vi "Ball Target Loop.vi"(0 "Camera List":string[](array[string]), 1 "Instance":i32) -> ()   [LabVIEW 2025]
uses:
  Camera Set Up/Ctrl/White Balance.ctl
  State Machine/Ball States.ctl
  State Machine/Ball Main CLuster.ctl
  <vilib>/vision/Image Controls.llb/IMAQ Image.ctl
  Camera Set Up/Event/Event Setup Types.ctl
  Steam Type.ctl
  <vilib>/Utility/config.llb/Read Key (String).vi
  <vilib>/Utility/config.llb/Write Key (String).vi
  <vilib>/Utility/config.llb/NI_LVConfig.lvlib
  <vilib>/vision/NI_Vision_Development_Module.lvlib
panel:
  in  "Running":bool
  in  "Timeout":u32
  in  "Main":T1(tab)
  out "Image":T2(plugin-control)
  out "Camera Name":string="cam0"
  out "Fule Distance":dbl[](array[numeric]) caption="Distance" format="%.1f"
  out "Fule Angle":dbl[](array[numeric]) caption="Angle" format="%.1f"
  in  "Settings":bool
  in  "Save":bool
  in  "Tools":bool
  out "Ball Fps":dbl format="%#.0f"
  in  "Color Range":T3={"Hue"={103, 151}, "Sat"={217, 255}, "Val"={201, 249}} {"Val" scale format="%#.0f"; "Sat" scale format="%#.0f"; "Hue" scale=0.0..255.0 scale format="%#.0f"}
  in  "Home":bool
  in  "Ball Diameter (in)":dbl=16.0
  in  "FOV":dbl=68.5
  out "Mask":T2(plugin-control)
  in  "Score Threshold %":dbl=80.0
  out "Camera Name 2":string="cam0"
  in  "VideoMode":u16(ring)=20 items=["160x120 MJPG 30.00fps", "160x120 YUY2 30.00fps", "176x144 MJPG 30.00fps", "176x144 YUY2 30.00fps", "320x240 MJPG 30.00fps", "320x240 YUY2 30.00fps", "352x288 MJPG 30.00fps", "352x288 YUY2 30.00fps", "416x240 MJPG 30.00fps", "424x240 YUY2 30.00fps", "640x360 MJPG 30.00fps", "640x360 YUY2 30.00fps", "640x480 MJPG 30.00fps", "640x480 YUY2 30.00fps", "800x448 MJPG 30.00fps", "800x448 YUY2 20.00fps", "800x600 MJPG 30.00fps", "800x600 YUY2 15.00fps", "960x544 MJPG 30.00fps", "960x544 YUY2 15.00fps", "1280x720 MJPG 30.00fps", "1280x720 YUY2 10.00fps", "1280x800 YUY2 10.00fps"]
  in  "Saturation":i32(slide)=50 min=1 max=100 scale=0.0..100.0
  in  "Hue":i32(slide)=50 min=1 max=100 scale=0.0..100.0
  in  "Gamma":i32(slide)=50 min=1 max=100 scale=0.0..100.0
  in  "Exposure":dbl(slide)=2.0 min=1.0 max=5.0 scale=0.0..5.0
  in  "Contrast":i32(slide)=50 min=1 max=100 scale=0.0..100.0
  in  "Sharpness":i32(slide)=50 min=1 max=100 scale=0.0..100.0
  in  "White Balance":T4=enum."Hold current"
  in  "Gain":i32(slide)=50 min=1 max=100 scale=0.0..100.0
  in  "Brightness":i32(slide)=50 min=1 max=100 scale=0.0..100.0
  in  "Save 2":bool caption="Save"
  out "Width":u32=640
  out "Height":u32=360
  out "Camera Name 3":string="cam0"
  in  "Home 2":bool caption="Home"
  out "Camera Image":T2(plugin-control)
  out "Data to Send":dbl[][](array[numeric])
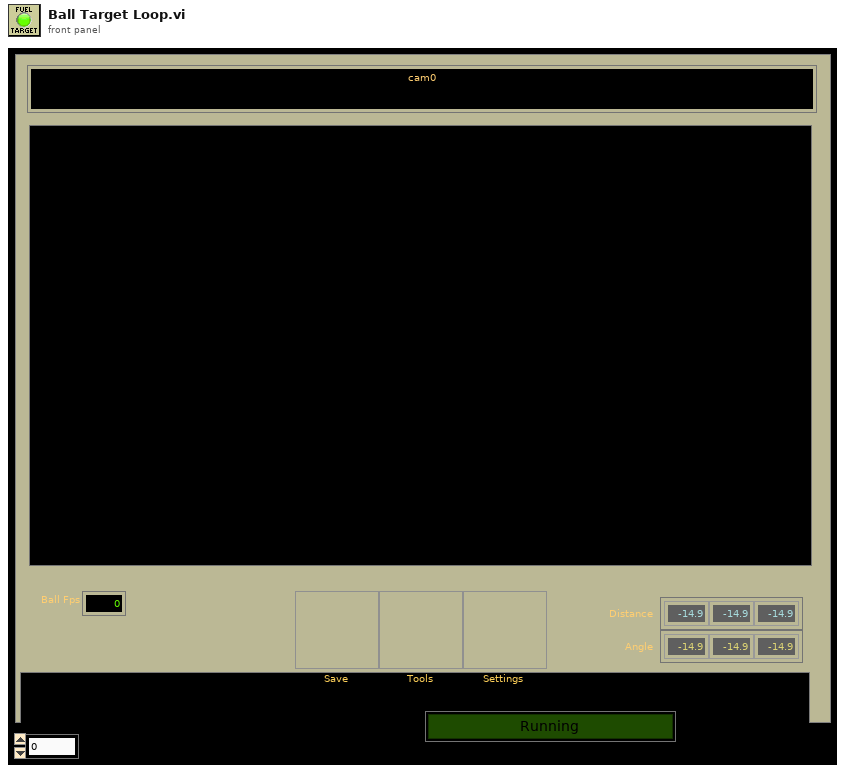
[diagram p1: front panel]
types:
  T1 = enum32{"Main", "Threshold", "Camera Settings", "Misc"}
  T2 = typedef "IMAQ Image.ctl" = refnum<image>
  T3 = cluster{"Hue":cluster{i64, i64}, "Sat":cluster{i64, i64}, "Val":cluster{i64, i64}}
  T4 = typedef "White Balance.ctl" = enum16{"Auto", "Fixed indoor", "Fixed outdoor 1", "Fixed outdoor 2", "Fixed fluorescent 1", "Fixed fluorescent 2", "Hold current", "Custom"}
  T5 = typedef "Ball Main CLuster.ctl" = cluster{"Ball FIFO":T6[], "Camera Name":string, "Ball path":path, "Control Ref's":refnum<vi>[], "Mask Image":T2, "Main Image":T2, "Algae Color Range":cluster{"Hue":cluster{dbl, dbl}, "Sat":cluster{dbl, dbl}, "Val":cluster{dbl, dbl}}, "EDIT Settings":bool, "Camera Number":i32}
  T6 = typedef "Ball States.ctl" = enum16{"Message Dispatcher", "INI", "Open", "Save", "Exit"}
  T7 = typedef "Particle Parameters" = i32
  T8 = typedef "Event Setup Types.ctl" = enum16{"Default", "Camera Loop Started", "GreyScale", "Reset Camera Settings", "Reset Team Number", "Save Data", "Setting Changed", "Update Video Mode", "Video Mode Changed", "Exit"}
  T9 = cluster{"Hue":cluster{dbl, dbl}, "Sat":cluster{dbl, dbl}, "Val":cluster{dbl, dbl}}
  T10 = cluster{"Hue":cluster{i64, dbl}, "Sat":cluster{i64, dbl}, "Val":cluster{i64, dbl}}
  T11 = typedef "Target Fields.ctl" = cluster{"diameter points":cluster{"first point":cluster{"x":dbl, "y":dbl}, "projected point":cluster{"x":dbl, "y":dbl}}, "normalized center":cluster{"x":dbl, "y":dbl}, "Overall Score":dbl, "Area Score":dbl, "Moment Score":dbl, "Aspect Score":dbl, "Distance (ft)":dbl, "Upper Goal":bool}
  T12 = cluster{cluster{"Lower":dbl, "Upper":dbl}, cluster{"Lower":dbl, "Upper":dbl}, cluster{"Lower":dbl, "Upper":dbl}}
  T13 = typedef "Image Type" = u32
  T14 = typedef "NI_LVConfig.lvlib/Config Data RefNum.ctl" = refnum<k1>
  T15 = typedef "Steam Type.ctl" = enum8{"Unknown", "Apriltag", "Fuel", "Other"}
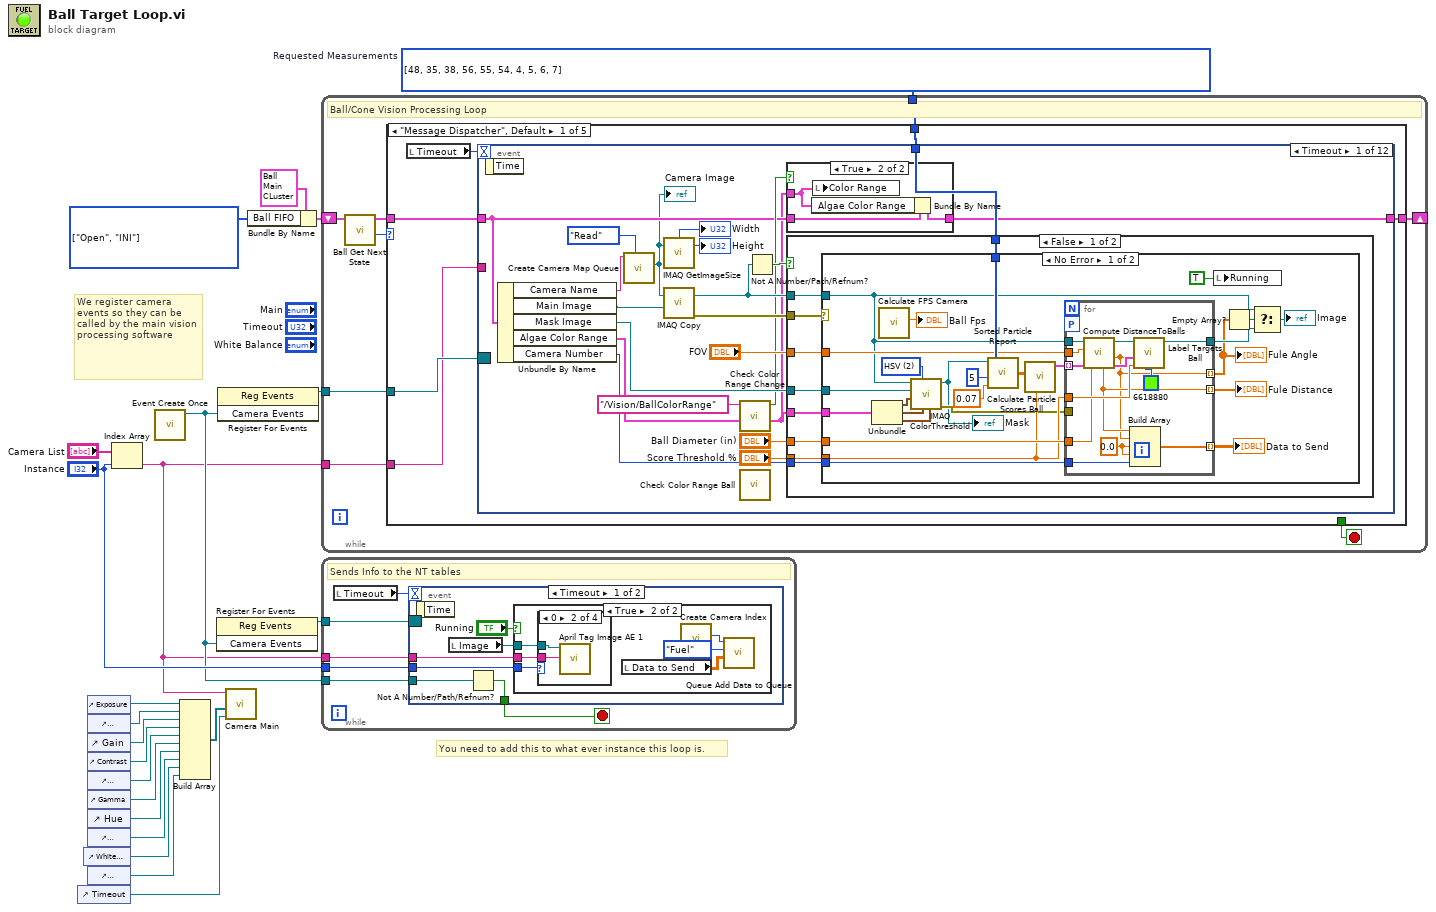
[diagram p0: block diagram]
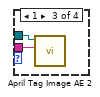
[diagram p4: hidden frame]
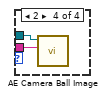
[diagram p5: hidden frame]
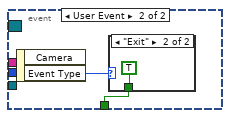
[diagram p6: hidden frame]
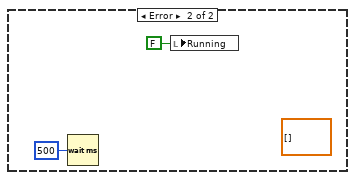
[diagram p9: hidden frame]
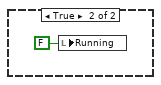
[diagram p10: hidden frame]
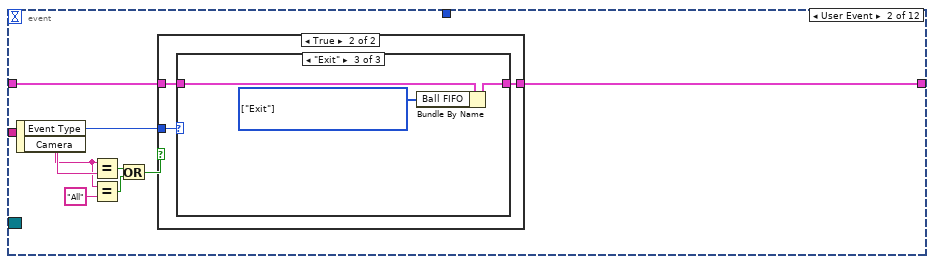
[diagram p11: hidden frame]
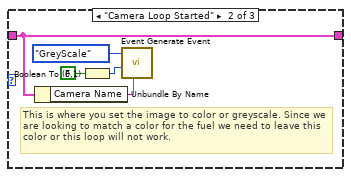
[diagram p14: hidden frame]
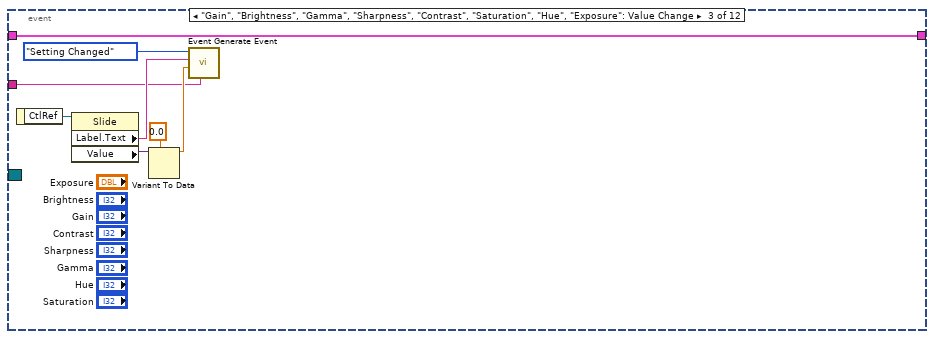
[diagram p15: hidden frame]
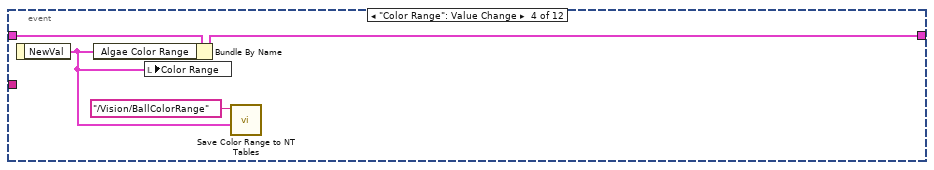
[diagram p16: hidden frame]
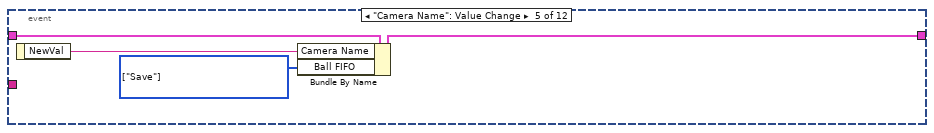
[diagram p17: hidden frame]
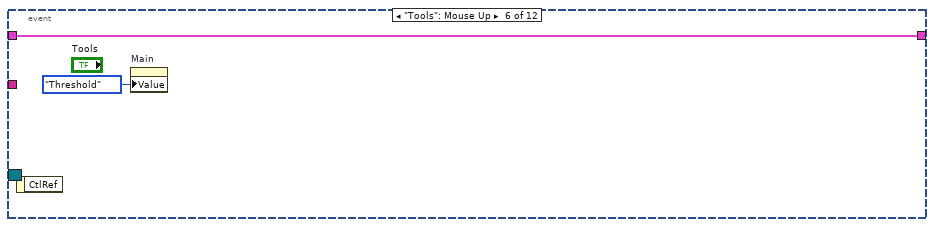
[diagram p18: hidden frame]
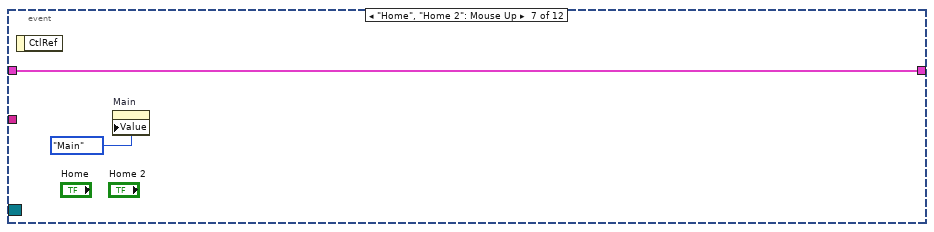
[diagram p19: hidden frame]
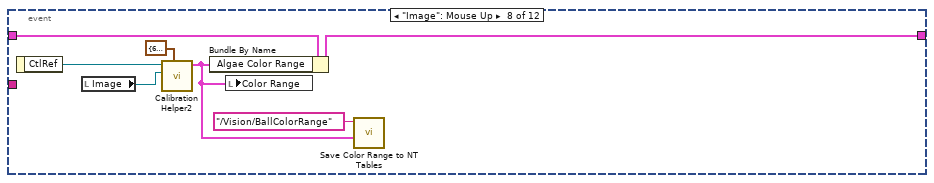
[diagram p20: hidden frame]
diagram:
  w19 = T6[] [enum."Open", enum."INI"] items=["Message Dispatcher", "INI", "Open", "Save", "Exit"] ("Ball FIFO")
  w21 = T7[] [48, 35, 38, 56, 55, 54, 4, 5, 6, 7] items=["Center of Mass X", "Center of Mass Y", "First Pixel X", "First Pixel Y", "Bounding Rect Left", "Bounding Rect Top", "Bounding Rect Right", "Bounding Rect Bottom", "Max Feret Diameter Start X", "Max Feret Diameter Start Y", "Max Feret Diameter End X", "Max Feret Diameter End Y", "Max Horiz. Segment Length Left", "Max Horiz. Segment Length Right", "Max Horiz. Segment Length Row", "-", "Bounding Rect Width", "Bounding Rect Height", "Bounding Rect Diagonal", "Perimeter", "Convex Hull Perimeter", "Holes' Perimeter", "Max Feret Diameter", "Equivalent Ellipse Major Axis", "Equivalent Ellipse Minor Axis", "Equivalent Ellipse Minor Axis (Feret)", "Equivalent Rect Long Side", "Equivalent Rect Short Side", "Equivalent Rect Diagonal", "Equivalent Rect Short Side (Feret)", "Average Horiz. Segment Length", "Average Vert. Segment Length", "Hydraulic Radius", "Waddel Disk Diameter", "-", "Area", "Holes' Area", "Particle & Holes' Area", "Convex Hull Area", "Image Area", "-", "Number of Holes", "Number of Horiz. Segments", "Number of Vert. Segments", "-", "Orientation", "Max Feret Diameter Orientation", "-", "% Area/Image Area", "% Area/(Particle & Holes' Area)", "Ratio of Equivalent Ellipse Axes", "Ratio of Equivalent Rect Sides", "-", "Elongation Factor", "Compactness Factor", "Heywood Circularity Factor", "Type Factor", "-", "Sum X", "Sum Y", "Sum XX", "Sum XY", "Sum YY", "Sum XXX", "Sum XXY", "Sum XYY", "Sum YYY", "-", "Moment of Inertia XX", "Moment of Inertia XY", "Moment of Inertia YY", "Moment of Inertia XXX", "Moment of Inertia XXY", "Moment of Inertia XYY", "Moment of Inertia YYY", "Norm. Moment of Inertia XX", "Norm. Moment of Inertia XY", "Norm. Moment of Inertia YY", "Norm. Moment of Inertia XXX", "Norm. Moment of Inertia XXY", "Norm. Moment of Inertia XYY", "Norm. Moment of Inertia YYY", "Hu Moment 1", "Hu Moment 2", "Hu Moment 3", "Hu Moment 4", "Hu Moment 5", "Hu Moment 6", "Hu Moment 7"]  # Requested Measurements
  # "You need to add this to what ever instance this loop is."
  # "We register camera events so they can be called by the main vision processing software"
  n1 = control-ref of="Timeout"() -> (w4:refnum<vi>)
  n2 = control-ref of="White Balance"() -> (w3:refnum<vi>)
  n3 = control-ref of="Exposure"() -> (w13:refnum<vi>)
  n4 = control-ref of="Brightness"() -> (w12:refnum<vi>)
  n5 = control-ref of="Gain"() -> (w11:refnum<vi>)
  n6 = control-ref of="Contrast"() -> (w10:refnum<vi>)
  n7 = control-ref of="Sharpness"() -> (w9:refnum<vi>)
  n8 = control-ref of="Gamma"() -> (w8:refnum<vi>)
  n9 = control-ref of="Hue"() -> (w7:refnum<vi>)
  n10 = control-ref of="Saturation"() -> (w6:refnum<vi>)
  n11 = control-ref of="VideoMode"() -> (w2:refnum<vi>)
  n12 = Index Array(array="Camera List", index="Instance") -> (element=w5:string)
  n13 = call "Event Create Once.vi"() -> ("Camera Events"=w14:refnum<user-event>)  [unwired: 10 in, 1 out]
  n14 = Build Array(w13, w12, w11, w10, w9, w8, w7, w6, w3, w2) -> (w1:refnum<vi>[])
  n15 = register-events(w14) -> (reference out=w15:refnum<event-registration>)  [unwired: 2 in, 1 out]
  n16 = register-events(w14) -> (reference out=w22:refnum<event-registration>)  [unwired: 2 in, 1 out]
  n17 = call "Camera Main.vi"("Timeout 2"=w4, "Main Open and Save Ctrls Ref"=w1, "Camera"=w5) -> ()  [unwired: 9 in]
  n18 = Bundle By Name(cluster=T5 {"Ball FIFO"=[], "Camera Name"="", "Ball path"=path "", "Control Ref's"=[], "Mask Image"=refnum, "Main Image"=refnum, "Algae Color Range"={"Hue"={21.620689392089844, 69.62068939208984}, "Sat"={66.41378784179688, 255.0}, "Val"={96.0, 255.0}}, "EDIT Settings"=FALSE, "Camera Number"=5} ("Ball Main Cluster in"), "Ball FIFO"=w19) -> (w20:T5)
  n19 = while {
    tunnel: w21 -> [w30]
    tunnel: w22 -> [w29]
    shift-right: [w24] -> _
    shift-left: w20 -> [w27]
    tunnel: w5 -> [w23]
    stop <- w28 stop-if-true
    # "Ball/Cone Vision Processing Loop"
    n20 = call "Ball Get Next State.vi"("Ball Main Cluster in"=w27) -> ("Next State"=w26:T6, "Ball Main Cluster out"=w25:T5)  [unwired: 9 in]
    n21 = case shown="\"Message Dispatcher\", Default" w26 {
      tunnel: w30 -> [w36 _ _ _ _]
      tunnel: w29 -> [w35 _ _ _ _]
      tunnel: [_ _ _ _ TRUE] -> w28
      tunnel: w25 -> [w33 w191 w205 w258 w275]
      tunnel: [w34 w190 w203 w258 w275] -> w24
      tunnel: w23 -> [w31 w175 _ _ _]
      frame "Message Dispatcher", Default {
        n22 = local read "Timeout"() -> (w32:u32)
        n23 = event shown="[0] Timeout" {
          selector: w35 -> [_ _ _ _ _ _ _ _ _ _ _ _]
          dyn-events: _ -> [_ _ _ _ _ _ _ _ _ _ _ _]
          timeout: w32 -> [_ _ _ _ _ _ _ _ _ _ _ _]
          tunnel: w36 -> [w57 _ _ _ _ _ _ _ _ _ _ _]
          tunnel: w33 -> [w43 w122 w136 w147 w151 w153 w155 w159 w165 w167 w170 w174]
          tunnel: [w41 w120 w136 w146 w150 w153 w155 w158 w164 w167 w170 w174] -> w34
          tunnel: w31 -> [_ w118 w137 _ _ _ _ _ _ w166 _ w173]
          event Timeout {
            n24 = event-data() -> ()  [unwired: 1 in, 1 out]
            n25 = Unbundle By Name(w43) -> ("Camera Name"=w56:string, "Main Image"=w54:T2, "Mask Image"=w55:T2, "Algae Color Range"=w45:T9, "Camera Number"=w40:i32)
            n26 = call "Create Camera Map Queue.vi"("Action"=enum16{"Read", "Write"}."Read", "Camera"=w56) -> ("Image out"=w37:T2)  [unwired: 8 in, 1 out]
            "Camera Image" <- w37
            n27 = call "IMAQ GetImageSize"("Image"=w37) -> ("Y Resolution"=→"Height":i32, "X Resolution"=→"Width":i32)  [unwired: 3 in, 1 out]
            n28 = call "IMAQ Copy"("Image Dst"=w54, "Image Src"=w37) -> ("error out"=w49:errorcluster, "Image Dst Out"=w47:T2)  [unwired: 4 in]
            n29 = call "Check Color Range Change.vi"("Color Range in"=w45, "Name"="/Vision/BallColorRange") -> ("Color Range out"=w42:T10, "Changed"=w46:bool)  [unwired: 8 in]
            n30 = call "Check Color Range Ball.vi"() -> ()  [unwired: 12 in]
            n31 = Not A Number/Path/Refnum?(number/path/refnum=w47) -> (NaN/Path/Refnum?=w48:bool)
            n32 = case shown="True" w46 {
              tunnel: w42 -> [_ w59]
              tunnel: w43 -> [w58 w61]
              tunnel: [w58 w60] -> w41
              frame False {
              }
              frame True {
                n33 = Bundle By Name(cluster=w61, "Algae Color Range"=w59) -> (w60:T5)
                n34 = local write "Color Range"(w59) -> ()
              }
            }
            n35 = case shown="False" w48 {
              tunnel: w57 -> [w70 _]
              tunnel: w55 -> [w69 _]
              tunnel: w42 -> [w68 _]
              tunnel: "Ball Diameter (in)" -> [w67 _]
              tunnel: "Score Threshold %" -> [w66 _]
              tunnel: "FOV" -> [w65 _]
              tunnel: w47 -> [w64 _]
              tunnel: w49 -> [w63 _]
              tunnel: w40 -> [w62 _]
              frame False {
                n36 = case shown="No Error" w63 {
                  tunnel: w70 -> [w96 _]
                  tunnel: w69 -> [w94 _]
                  tunnel: w65 -> [w93 _]
                  tunnel: w68 -> [w92 _]
                  tunnel: w67 -> [w91 _]
                  tunnel: w66 -> [w90 _]
                  tunnel: w64 -> [w76 _]
                  tunnel: w62 -> [w72 _]
                  frame No Error {
                    w85 = u16 2 items=["RGB", "HSL", "HSV", "HSI"] ("Color Mode")
                    n37 = Unbundle(w92) -> ("Hue"=w81:cluster{i64, dbl}, "Sat"=w80:cluster{i64, dbl}, "Val"=w79:cluster{i64, dbl})
                    n38 = call "Calculate FPS Camera.vi"() -> ("Fps"=→"Ball Fps":dbl)  [unwired: 11 in]
                    n39 = call "IMAQ ColorThreshold"("Blue or Luma or Val or Inten Range"=w79, "Green or Sat Range"=w80, "Color Mode"=w85, "Red or Hue Range"=w81, "Image Dst"=w94, "Image Src"=w76) -> ("error out"=w84:errorcluster, "Image Dst Out"=w77:T2)  [unwired: 4 in]
                    "Mask" <- w77
                    n40 = call "Sorted Particle Report.vi"("Min Area Size %"=0.07 ("Size Limit %"), "Particle Count Limit"=5 ("Particle Count LImit"), "Pixel Measurements"=w96, "Image in"=w77) -> ("Sorted Data"=w88:dbl[][])  [unwired: 2 out]
                    n41 = call "Calculate Particle Scores Ball.vi"("Limit"=w90, "Sorted Data"=w88) -> ("Scores"=w87:T11[])  [unwired: 9 in]
                    n42 = for {
                      tunnel: w87 -> [w108] mode=indexing
                      tunnel: w90 -> [w109]
                      tunnel: [w98] -> w75 mode=indexing
                      tunnel: w84 -> [_]
                      tunnel: w93 -> [w104]
                      tunnel: [w99] -> w74 mode=indexing
                      tunnel: w91 -> [w102]
                      tunnel: [w100] -> w73 mode=indexing
                      workers-P: _ -> [_]
                      tunnel: w76 -> [w106]
                      tunnel: [w110] -> w83
                      tunnel: w72 -> [w97]
                      w101 = 0.0 ("element")
                      n43 = call "Compute DistanceToBalls.vi"("Target Width (in)"=w102, "results"=w108, "FOV"=w104, "Image Src"=w106) -> ("results out"=w105:T11, "Off Angle"=w98:dbl, "Image Dst Out"=w107:T2, "Distance"=w99:dbl)  [unwired: 4 in]
                      n44 = Build Array(w99, w98, w101, w101, w97) -> (w100:dbl[])
                      n45 = call "Label Targets Ball.vi"("Color"=u32 6618880, "Score Threshold"=w109, "results"=w105, "Angle"=w98, "Image in"=w107) -> ("Image out"=w110:T2)  [unwired: 6 in]
                    }
                    "Fule Angle" <- w75
                    "Fule Distance" <- w74
                    "Data to Send" <- w73
                    n46 = local write "Running"(TRUE ("Running")) -> ()
                    n47 = Empty Array?(array=w75) -> (empty?=w82:bool)
                    n48 = Select(t=w76, s=w82, f=w83) -> (s? t:f=→"Image":T2)
                  }
                  frame Error {
                    (unwired) dbl[][] []
                    n49 = Wait (ms)(milliseconds to wait=u32 500) -> ()  [unwired: 1 out]
                    n50 = local write "Running"(FALSE ("Running")) -> ()
                  }
                }
              }
              frame True {
                n51 = local write "Running"(FALSE ("Running")) -> ()
              }
            }
          }
          event User Event {
            n52 = event-data() -> ("Event Type"=w121:T8, "Camera"=w115:string)  [unwired: 1 in]
            n53 = Equal?(x=w115, y=w118) -> (x = y?=w117:bool)
            n54 = Equal?(x=w115, y="All") -> (x = y?=w116:bool)
            n55 = Or(x=w117, y=w116) -> (x .or. y?=w114:bool)
            n56 = case shown="True" w114 {
              tunnel: w122 -> [w123 w126]
              tunnel: w121 -> [_ w125]
              tunnel: [w123 w124] -> w120
              frame False {
              }
              frame True {
                n57 = case shown="\"Exit\"" w125 {
                  tunnel: w126 -> [w127 w128 w135]
                  tunnel: [w127 w128 w134] -> w124
                  frame "Default", Default {
                  }
                  frame "Camera Loop Started" {
                    # "This is where you set the image to color or greyscale. Since we are looking to match a color for the fuel we need to leave this color or this loop will not work."
                    n58 = Unbundle By Name(w128) -> ("Camera Name"=w131:string)
                    n59 = Boolean To (0,1)(Boolean=FALSE) -> (0, 1=w132:i16)
                    n60 = call "Event Generate Event.vi"("Camera Name"=w131, "Setpoint"=w132, "Event Type"=Event_Setup_Types."GreyScale") -> ()  [unwired: 9 in]
                  }
                  frame "Exit" {
                    w133 = T6[] [enum."Exit"] items=["Message Dispatcher", "INI", "Open", "Save", "Exit"] ("Ball FIFO")
                    n61 = Bundle By Name(cluster=w135, "Ball FIFO"=w133) -> (w134:T5)
                  }
                }
              }
            }
          }
          event "Gain", "Brightness", "Gamma", "Sharpness", "Contrast", "Saturation", "Hue", "Exposure": Value Change {
            n62 = event-data() -> ("CtlRef"=w138:refnum<vi>)  [unwired: 1 in]
            n63 = property on="Property Node" class="Slide"(reference=w138) -> ("Label.Text"=w142:string, "Value"=w141:variant)  [unwired: 1 in, 2 out]
            n64 = Variant To Data(type=0.0, Variant=w141) -> (data=w139:dbl)  [unwired: 1 in, 1 out]
            n65 = call "Event Generate Event.vi"("Camera Name"=w137, "Setpoint"=w139, "Setting Name"=w142, "Event Type"=Event_Setup_Types."Setting Changed") -> ()  [unwired: 8 in]
          }
          event "Color Range": Value Change {
            n66 = event-data() -> ("NewVal"=w144:T3)  [unwired: 1 in]
            n67 = Bundle By Name(cluster=w147, "Algae Color Range"=w144) -> (w146:T5)
            n68 = local write "Color Range"(w144) -> ()
            n69 = call "Save Color Range to NT Tables.vi"("Color Range"=w144, "Color Range Name"="/Vision/BallColorRange") -> ()  [unwired: 8 in, 2 out]
          }
          event "Camera Name": Value Change {
            w148 = T6[] [enum."Save"] items=["Message Dispatcher", "INI", "Open", "Save", "Exit"] ("Ball FIFO")
            n70 = event-data() -> ("NewVal"=w149:string)  [unwired: 1 in]
            n71 = Bundle By Name(cluster=w151, "Camera Name"=w149, "Ball FIFO"=w148) -> (w150:T5)
          }
          event "Tools": Mouse Up {
            n72 = event-data() -> ()  [unwired: 1 in, 1 out]
            n73 = property on="Main" class="TabCtl (strict)"("Value"=T1."Threshold" ("Main")) -> ()  [unwired: 2 in, 2 out]
          }
          event "Home", "Home 2": Mouse Up {
            n74 = event-data() -> ()  [unwired: 1 in, 1 out]
            n75 = property on="Main" class="TabCtl (strict)"("Value"=T1."Main" ("Main")) -> ()  [unwired: 2 in, 2 out]
          }
          event "Image": Mouse Up {
            n76 = event-data() -> ("CtlRef"=w161:refnum<vi>)  [unwired: 1 in]
            n77 = local read "Image"() -> (w160:T2)
            n78 = call "Calibration Helper2.vi"("Std Devs"=cluster{"H":dbl, "S":dbl, "V":dbl} {"H"=6.0, "S"=6.0, "V"=6.0} ("Std Devs Ball"), "Image"=w160, "Image Ctl Refnum"=w161) -> ("output color"=w156:T12)  [unwired: 7 in, 1 out]
            n79 = Bundle By Name(cluster=w159, "Algae Color Range"=w156) -> (w158:T5)
            n80 = local write "Color Range"(w156) -> ()
            n81 = call "Save Color Range to NT Tables.vi"("Color Range"=w156, "Color Range Name"="/Vision/BallColorRange") -> ()  [unwired: 8 in, 2 out]
          }
          event "Save": Mouse Up {
            w163 = T6[] [enum."Save"] items=["Message Dispatcher", "INI", "Open", "Save", "Exit"] ("Ball FIFO")
            n82 = event-data() -> ()  [unwired: 1 in, 1 out]
            n83 = Bundle By Name(cluster=w165, "Ball FIFO"=w163) -> (w164:T5)
          }
          event "Save 2": Mouse Up {
            n84 = event-data() -> ()  [unwired: 1 in, 1 out]
            n85 = call "Event Generate Event.vi"("Camera Name"=w166, "Event Type"=Event_Setup_Types."Save Data") -> ()  [unwired: 10 in]
          }
          event "Settings": Mouse Up {
            n86 = event-data() -> ()  [unwired: 1 in, 1 out]
            n87 = property on="Main" class="TabCtl (strict)"("Value"=T1."Camera Settings" ("Main")) -> ()  [unwired: 2 in, 2 out]
          }
          event "VideoMode": Value Change {
            n88 = event-data() -> ("NewVal"=w172:u16)  [unwired: 1 in]
            n89 = call "Event Generate Event.vi"("Camera Name"=w173, "Setpoint"=w172, "Event Type"=Event_Setup_Types."Video Mode Changed") -> ()  [unwired: 9 in]
          }
        }
      }
      frame "INI" {
        w188 = T13 4 items=["Grayscale (U8)", "Grayscale (I16)", "Grayscale (SGL)", "Complex (CSG)", "RGB (U32)", "HSL (U32)", "RGB (U64)", "Grayscale (U16)"] ("Image Type")
        w192 = T13 0 items=["Grayscale (U8)", "Grayscale (I16)", "Grayscale (SGL)", "Complex (CSG)", "RGB (U32)", "HSL (U32)", "RGB (U64)", "Grayscale (U16)"] ("Image Type")
        n90 = call "Event Generate Event.vi"("Camera Name"=w175, "Setpoint"=i64 0, "Event Type"=Event_Setup_Types."GreyScale") -> ()  [unwired: 9 in]
        n91 = Match Pattern(string=w175, regular expression="[1-9]") -> (match substring=w178:string)  [unwired: 1 in, 3 out]
        n92 = Concatenate Strings(w175, "Algae Mask" ("string")) -> (w194:string)
        n93 = Concatenate Strings(w175, "Ball Main" ("string")) -> (w187:string)
        n94 = Fract/Exp String To Number(string=w178, default (0 dbl)=u32 0 ("default (0 DBL)")) -> (number=w177:u32)  [unwired: 2 in, 1 out]
        n95 = call "IMAQ Create"("Image Name"=w194, "Image Type"=w192) -> ("New Image"=w189:T2)  [unwired: 2 in, 2 out]
        n96 = call "IMAQ Create"("Image Name"=w187, "Image Type"=w188) -> ("New Image"=w185:T2)  [unwired: 2 in, 2 out]
        n97 = call "Save Color Range to NT Tables.vi"("Color Range"="Color Range", "Color Range Name"="/Vision/BallColorRange") -> ()  [unwired: 8 in, 2 out]
        n98 = Bundle By Name(cluster=w191, "Camera Name"=w175, "Mask Image"=w189, "Algae Color Range"="Color Range", "Main Image"=w185, "EDIT Settings"=FALSE, "Camera Number"=w177) -> (w190:T5)
        "Camera Name" <- w175
        "Camera Name 2" <- w175
        "Camera Name 3" <- w175
      }
      frame "Open" {
        n99 = call <vilib>:"Application Directory.vi"() -> ("Application Directory"=w208:path)
        n100 = Concatenate Strings("Ball" ("string"), ".ini" ("name or relative path")) -> (w220:string)
        n101 = Build Path(base path=w208, name or relative path="Config") -> (appended path=w206:path)
        n102 = Build Path(base path=w206, name or relative path=w220) -> (appended path=w201:path)
        n103 = control-ref of="Main"() -> (w214:refnum<vi>)
        n104 = call <vilib>:"Check if File or Folder Exists.vi"("path"=w201) -> ("error out"=w197:errorcluster, "file or folder exists?"=w199:bool, "dup path"=w200:path)  [unwired: 8 in]
        n105 = control-ref of="Color Range"() -> (w195:refnum<vi>)
        n106 = control-ref of="Ball Diameter (in)"() -> (w213:refnum<vi>)
        n107 = control-ref of="FOV"() -> (w212:refnum<vi>)
        n108 = control-ref of="Score Threshold %"() -> (w211:refnum<vi>)
        n109 = control-ref of="Camera Name"() -> (w196:refnum<vi>)
        n110 = case shown="True" w199 {
          tunnel: [w223 w224] -> w209
          tunnel: w200 -> [w222 w225]
          tunnel: [w222 w225] -> w198
          tunnel: w197 -> [w221 w224]
          frame False {
            n111 = call <vilib>:"Create File and Containing Folders.vi"("error in (no error)"=w221, "file path"=w222) -> ("error out"=w223:errorcluster)  [unwired: 8 in, 1 out]
          }
          frame True {
          }
        }
        n112 = Build Array(w195, w214, w213, w212, w211, w196) -> (w202:refnum<vi>[])
        n113 = call <vilib>:"Open Config Data.vi"("error in (no error)"=w209, "configuration file path"=w198) -> ("error out"=w215:errorcluster, "refnum"=w219:T14)  [unwired: 7 in, 1 out]
        n114 = for {
          tunnel: "Info" ("Camera Name") -> [w238]
          tunnel: w202 -> [w228] mode=indexing
          shift-right: [w240] -> w218
          shift-left: w219 -> [w241]
          shift-right: [w239] -> w217
          shift-left: w215 -> [w237]
          n115 = property on="Property Node" class="Ctl"(reference=w228) -> (reference out=w234:refnum<vi>, error out=w233:errorcluster, "Label.Text"=w231:string, "Value"=w227:variant)  [unwired: 1 in]
          n116 = Variant To Flattened String(Variant=w227) -> (data string=w229:string, 1:w226:i16[])
          n117 = call-poly <vilib>:"Read Key.vi"("section"=w238, "error in (no error)"=w237, "key"=w231, "refnum"=w241) -> ("error out"=w230:errorcluster, "value"=w235:string, "found?"=w236:bool, "refnum out"=w232:T14)  [unwired: 4 in]
          n118 = case shown="True" w236 {
            tunnel: w235 -> [_ w250]
            tunnel: w234 -> [_ w255]
            tunnel: w233 -> [_ w254]
            tunnel: w232 -> [w248 w253]
            tunnel: w238 -> [w247 _]
            tunnel: w231 -> [w246 _]
            tunnel: [w245 w253] -> w240
            tunnel: w230 -> [w244 w252]
            tunnel: [w243 w252] -> w239
            tunnel: w229 -> [w242 _]
            tunnel: w226 -> [_ w249]
            frame False {
              n119 = call-poly <vilib>:"Write Key.vi"("section"=w247, "error in (no error)"=w244, "value"=w242, "key"=w246, "refnum"=w248) -> ("error out"=w243:errorcluster, "refnum out"=w245:T14)  [unwired: 4 in, 1 out]
            }
            frame True {
              n120 = Flattened String To Variant(6:w250, 7:w249) -> (3:w251:variant)  [unwired: 1 in, 1 out]
              n121 = property on="Property Node" class="Ctl"(reference=w255, error in=w254, "Value"=w251) -> ()  [unwired: 2 out]
            }
          }
        }
        n122 = call <vilib>:"Close Config Data.vi"("error in (no error)"=w217, "refnum"=w218) -> ()  [unwired: 8 in, 2 out]
        n123 = Bundle By Name(cluster=w205, "Control Ref's"=w202, "Ball path"=w198) -> (w203:T5)
      }
      frame "Save" {
        n124 = Unbundle By Name(w258) -> ("Control Ref's"=w256:refnum<vi>[], "Ball path"=w257:path)
        n125 = call <vilib>:"Open Config Data.vi"("configuration file path"=w257) -> ("error out"=w262:errorcluster, "refnum"=w263:T14)  [unwired: 8 in, 1 out]
        n126 = for {
          tunnel: w256 -> [w273] mode=indexing
          tunnel: w263 -> [w272]
          tunnel: w262 -> [w271]
          tunnel: "Info" ("Camera Name") -> [w267]
          tunnel: [w265] -> w261
          tunnel: [w264] -> w260
          n127 = property on="Property Node" class="Ctl"(reference=w273, error in=w271) -> (error out=w268:errorcluster, "Label.Text"=w270:string, "Value"=w269:variant)  [unwired: 1 out]
          n128 = Variant To Flattened String(Variant=w269) -> (data string=w266:string)  [unwired: 1 out]
          n129 = call-poly <vilib>:"Write Key.vi"("section"=w267, "error in (no error)"=w268, "value"=w266, "key"=w270, "refnum"=w272) -> ("error out"=w265:errorcluster, "refnum out"=w264:T14)  [unwired: 4 in, 1 out]
        }
        n130 = call <vilib>:"Close Config Data.vi"("error in (no error)"=w261, "refnum"=w260) -> ()  [unwired: 8 in, 2 out]
      }
      frame "Exit" {
        n131 = Unbundle By Name(w275) -> ("Mask Image"=w277:T2, "Main Image"=w276:T2)
        n132 = call "IMAQ Dispose"("Image"=w277) -> ()  [unwired: 5 in, 1 out]
        n133 = call "IMAQ Dispose"("Image"=w276) -> ()  [unwired: 5 in, 1 out]
      }
    }
  }
  n134 = while {
    tunnel: w15 -> [w283]
    tunnel: "Instance" -> [w281]
    tunnel: w5 -> [w280]
    tunnel: w14 -> [w279]
    stop <- w282 stop-if-true
    # "Sends Info to the NT tables"
    n135 = local read "Timeout"() -> (w278:u32)
    n136 = event shown="[0] Timeout" {
      selector: w283 -> [_ _]
      dyn-events: _ -> [_ _]
      timeout: w278 -> [_ _]
      tunnel: [w285 w302] -> w282
      tunnel: w281 -> [w288 _]
      tunnel: w280 -> [w287 _]
      tunnel: w279 -> [w286 _]
      event Timeout {
        n137 = event-data() -> ()  [unwired: 1 in, 1 out]
        n138 = local read "Image"() -> (w289:T2)
        n139 = Not A Number/Path/Refnum?(number/path/refnum=w286) -> (NaN/Path/Refnum?=w285:bool)
        n140 = case shown="True" "Running" {
          tunnel: w289 -> [_ w295]
          tunnel: w288 -> [_ w294]
          tunnel: w287 -> [_ w292]
          frame False {
          }
          frame True {
            n141 = case shown="0" w294 {
              tunnel: w295 -> [_ w297 w299 w301]
              tunnel: w292 -> [_ w296 w298 w300]
              frame Default {
              }
              frame 0 {
                n142 = call "April Tag Image AE 1.vi"("Camera Name"=w296, "Apriltag Image in"=w297) -> ()  [unwired: 9 in, 1 out]
              }
              frame 1 {
                n143 = call "April Tag Image AE 2.vi"("Camera Name"=w298, "Apriltag Image in"=w299) -> ()  [unwired: 9 in, 1 out]
              }
              frame 2 {
                n144 = call "AE Camera Ball Image.vi"("Camera Name"=w300, "Fuel Image in"=w301) -> ()  [unwired: 9 in, 1 out]
              }
            }
            n145 = local read "Data to Send"() -> (w293:dbl[][])
            n146 = call "Create Camera Index.vi"() -> ("Connection Ref"=w290:i32)  [unwired: 11 in]
            n147 = call "Queue Add Data to Queue.vi"("Target Info in"=w293, "Stream Type"=Steam_Type."Fuel", "Camera Index"=w290) -> ()  [unwired: 9 in]
          }
        }
      }
      event User Event {
        n148 = event-data() -> ("Event Type"=w303:T8)  [unwired: 1 in, 1 out]
        n149 = case shown="\"Exit\"" w303 {
          tunnel: [_ TRUE] -> w302
          frame Default {
          }
          frame "Exit" {
          }
        }
      }
    }
  }
